vi "Change Insert VI.vi"(7 "Abort Original VI":bool=TRUE, 8 "error in":errorcluster caption="错误输入（无错误）", 10 "Data":variant, 11 "PanelRootNode in":refnum<class "PanelRootNode.lvclass"> caption="DNL_LabVIEW Object in") -> (0 "error out":errorcluster caption="错误输出", 3 "PanelRootNode out":refnum<class "PanelRootNode.lvclass"> caption="DNL_LabVIEW Object out")   [LabVIEW 2016, in "PanelRootNode.lvclass"]
uses:
  PanelRootNode.lvclass
  C:/Users/CL/Desktop/ZcDAQprj0811/ZcDAQprj/Modules/DAQ-Display/PanelSplitToolkit/PanelLinkNode/PanelLinkNode.lvclass
  PanelObject/PanelObject.lvclass
  PanelLinkNode/PanelLinkNode.lvclass/PanelLinkNode.ctl
  PanelDataNode/PanelDataNode.lvclass
  PanelLinkNode/PanelLinkNode.lvclass
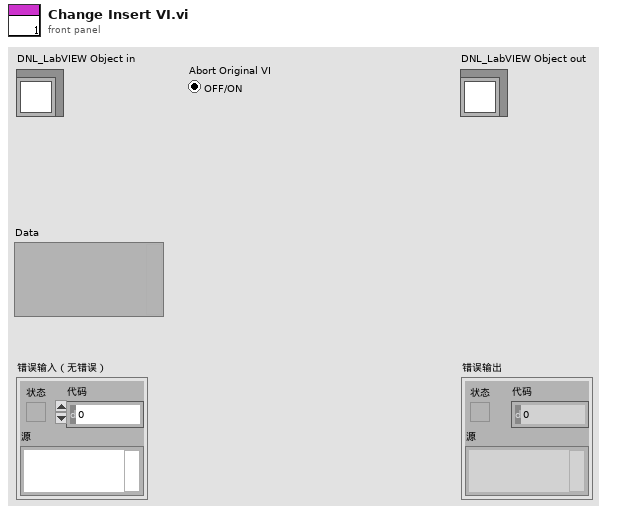
[diagram p1: front panel]
types:
  T1 = cluster{"Node*":refnum<data-value>, "VI*":refnum<vi>}
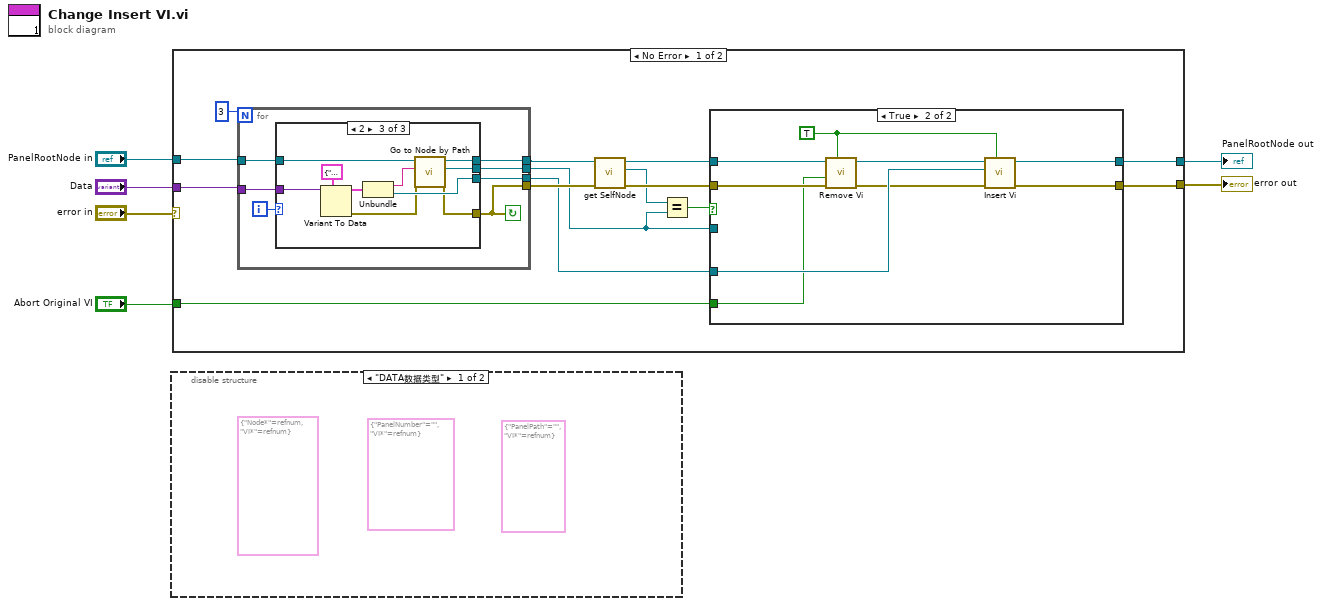
[diagram p0: block diagram]
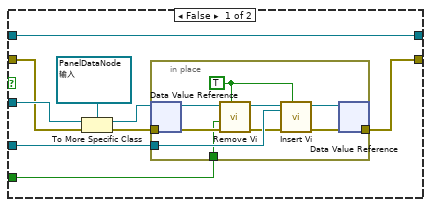
[diagram p3: hidden frame]
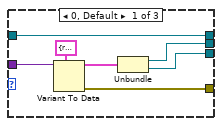
[diagram p4: hidden frame]
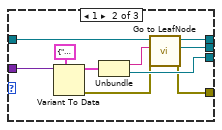
[diagram p5: hidden frame]
diagram:
  n1 = disable-structure shown="\"DATA数据类型\"" {
    frame condition #0 {
      (unwired) cluster{"PanelPath":string, "VI*":refnum<vi>} {"PanelPath"="", "VI*"=refnum}
      (unwired) cluster{"PanelNumber":string, "VI*":refnum<vi>} {"PanelNumber"="", "VI*"=refnum}
      (unwired) T1 {"Node*"=refnum, "VI*"=refnum}
    }
    frame condition #1 (active) {
    }
  }
  n2 = case shown="No Error" "error in" {
    selector: "error in" -> [_ w83]
    tunnel: [w8 w83] -> w3
    tunnel: [w9 w82] -> w1
    tunnel: "PanelRootNode in" -> [w20 w82]
    tunnel: "Data" -> [w18 _]
    tunnel: "Abort Original VI" -> [w7 _]
    frame No Error {
      n3 = for {
        N: 3 -> [_]
        tunnel: [w53] -> w13
        tunnel: [w52] -> w11
        tunnel: w20 -> [w51]
        tunnel: [w50] -> w10
        tunnel: [w49] -> w12
        tunnel: w18 -> [w48]
        i -> [w54]
        stop <- w49 continue-if-true
        n4 = case shown="2" w54 {
          tunnel: [w61 w71 w81] -> w50
          tunnel: [w60 w67 w77] -> w52
          tunnel: [w57 w69 w79] -> w53
          tunnel: [w58 w66 w76] -> w49
          tunnel: w51 -> [w57 w64 w75]
          tunnel: w48 -> [w56 w63 w73]
          frame 0, Default {
            n5 = Variant To Data(type=T1 {"Node*"=refnum, "VI*"=refnum}, Variant=w56) -> (data=w59:T1, error out=w58:errorcluster)  [unwired: 1 in]
            n6 = Unbundle(w59) -> ("Node*"=w60:refnum<data-value>, "VI*"=w61:refnum<vi>)
          }
          frame 1 {
            n7 = Variant To Data(type=cluster{"PanelNumber":string, "VI*":refnum<vi>} {"PanelNumber"="", "VI*"=refnum}, Variant=w63) -> (data=w70:cluster{"PanelNumber":string, "VI*":refnum<vi>}, error out=w65:errorcluster)  [unwired: 1 in]
            n8 = Unbundle(w70) -> ("PanelNumber"=w68:string, "VI*"=w71:refnum<vi>)
            n9 = call-dynamic "Go to LeafNode.vi"("error in"=w65, "LeafNumber"=w68, "PanelRootNode 输入"=w64) -> ("error out"=w66:errorcluster, "Node*"=w67:refnum<data-value>, "PanelRootNode 输出"=w69:refnum<class "PanelRootNode.lvclass">)  [unwired: 5 in, 1 out]
          }
          frame 2 {
            n10 = Variant To Data(type=cluster{"PanelPath":string, "VI*":refnum<vi>} {"PanelPath"="", "VI*"=refnum}, Variant=w73) -> (data=w80:cluster{"PanelPath":string, "VI*":refnum<vi>}, error out=w74:errorcluster)  [unwired: 1 in]
            n11 = Unbundle(w80) -> ("PanelPath"=w78:string, "VI*"=w81:refnum<vi>)
            n12 = call-dynamic "Go to Node by Path.vi"("error in"=w74, "NodePath"=w78, "PanelLinkNode 输入"=w75) -> ("error out"=w76:errorcluster, "Node*"=w77:refnum<data-value>, "PanelLinkNode 输出"=w79:refnum<class "PanelRootNode.lvclass">)  [unwired: 5 in, 1 out]
          }
        }
      }
      n13 = call "get SelfNode.vi"("error in (no error)"=w12, "PanelLinkNode输入"=w13) -> ("error out"=w17:errorcluster, "SelfNode*"=w14:refnum<data-value>, "PanelLinkNode输出"=w16:refnum<class "PanelRootNode.lvclass">)  [unwired: 7 in]
      n14 = Equal?(x=w14, y=w11) -> (x = y?=w15:bool)
      n15 = case shown="True" w15 {
        tunnel: w16 -> [w22 w44]
        tunnel: w10 -> [w29 w47]
        tunnel: [w22 w46] -> w9
        tunnel: w17 -> [w24 w42]
        tunnel: w11 -> [w26 _]
        tunnel: [w28 w45] -> w8
        tunnel: w7 -> [w21 w39]
        frame False {
          n16 = To More Specific Class(target class=refnum<data-value> refnum ("数据值引用"), reference=w26, error in=w24) -> (specific class reference=w25:refnum<data-value>, error out=w23:errorcluster)
          n17 = in-place {
            in-place-border: w29 -> [w38]
            in-place-border: w23 -> [w35]
            in-place-border: [w36] -> w28
            in-place-border: w21 -> [w30]
            w31 = TRUE ("Maintain ViValue(F)")
            n18 = in-place-dvr #1(w25) -> (w33:refnum<class "PanelDataNode.lvclass">)  [unwired: 1 out]
            n19 = call-dynamic "Remove Vi.vi"("Maitiain Vivalue(F)"=w31, "error in"=w35, "Abort VI"=w30, "PanelDataNode 输入"=w33) -> ("error out"=w34:errorcluster, "PanelDataNode 输出"=w32:refnum<class "PanelDataNode.lvclass">)  [unwired: 4 in, 2 out]
            n20 = call-dynamic "Insert Vi.vi"("Maintain ViValue(F)"=w31, "error in (no error)"=w34, "VI*"=w38, "PanelDataNode 输入"=w32) -> ("error out"=w36:errorcluster, "PanelDataNode 输出"=w37:refnum<class "PanelDataNode.lvclass">)  [unwired: 6 in]
            n21 = in-place-dvr #1(w37) -> ()  [unwired: 2 out]
          }
        }
        frame True {
          w40 = TRUE ("Maintain ViValue(F)")
          n22 = call-dynamic "Remove Vi.vi"("Maitiain Vivalue(F)"=w40, "error in"=w42, "Abort VI"=w39, "PanelDataNode 输入"=w44) -> ("error out"=w41:errorcluster, "PanelDataNode 输出"=w43:refnum<class "PanelRootNode.lvclass">)  [unwired: 4 in, 2 out]
          n23 = call-dynamic "Insert Vi.vi"("Maintain ViValue(F)"=w40, "error in (no error)"=w41, "VI*"=w47, "PanelDataNode 输入"=w43) -> ("error out"=w45:errorcluster, "PanelDataNode 输出"=w46:refnum<class "PanelRootNode.lvclass">)  [unwired: 6 in]
        }
      }
    }
    frame Error {
    }
  }
  "error out" <- w3
  "PanelRootNode out" <- w1
